vi "p20 codificador imagenes gris.vi"() -> ()   [LabVIEW 2013]
panel:
  in  "path to BMP file 2":path
  in  "path to BMP file":path
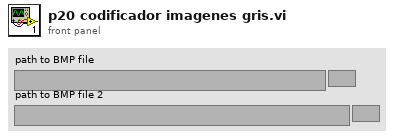
[diagram p1: front panel]
types:
  T1 = typedef "imagedata.ctl" = cluster{"image type":i32, "image depth":i32, "image":u8[], "mask":u8[], "colors":u32[], "Rectangle":cluster{"left":i16, "top":i16, "right":i16, "bottom":i16}}
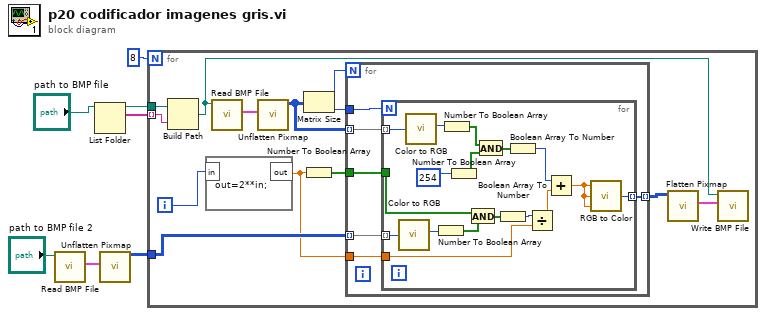
[diagram p0: block diagram]
diagram:
  n1 = call <vilib>:"Read BMP File.vi"("path to BMP file"="path to BMP file 2") -> ("image data"=w2:T1)  [unwired: 8 in, 2 out]
  n2 = List Folder(path="path to BMP file") -> (path out=w5:path, filenames=w4:string[])  [unwired: 3 in, 2 out]
  n3 = call <vilib>:"Unflatten Pixmap.vi"("image data"=w2) -> ("24-bit pixmap"=w1:u32[][])  [unwired: 4 in, 6 out]
  n4 = for {
    N: 8 -> [_]
    tunnel: w5 -> [w19]
    tunnel: w4 -> [w18] mode=indexing
    tunnel: w1 -> [w16]
    i -> [w20]
    n5 = Build Path(base path=w19, name or relative path=w18) -> (appended path=w13:path)
    n6 = formula code="out=2**in;"("in"=w20) -> ("out"=w12:dbl)
    n7 = call <vilib>:"Read BMP File.vi"("path to BMP file"=w13) -> ("image data"=w17:T1)  [unwired: 8 in, 2 out]
    n8 = call <vilib>:"Unflatten Pixmap.vi"("image data"=w17) -> ("24-bit pixmap"=w11:u32[][])  [unwired: 4 in, 6 out]
    n9 = Matrix Size(0:w11) -> (1:w9:i32, 2:w10:i32)
    n10 = Number To Boolean Array(number=w12) -> (Boolean array=w8:bool[])
    n11 = for {
      N: w9 -> [_]
      tunnel: w11 -> [w26] mode=indexing
      tunnel: w16 -> [w25] mode=indexing
      tunnel: [w24] -> w15 mode=indexing
      tunnel: w12 -> [w23]
      tunnel: w10 -> [w22]
      tunnel: w8 -> [w21]
      n12 = for {
        N: w22 -> [_]
        tunnel: w26 -> [w42] mode=indexing
        tunnel: w25 -> [w32] mode=indexing
        tunnel: [w28] -> w24 mode=indexing
        tunnel: w23 -> [w35]
        tunnel: w21 -> [w27]
        n13 = call <vilib>:"Color to RGB.vi"("Color"=w32) -> ("R"=w31:u8)  [unwired: 3 out]
        n14 = call <vilib>:"Color to RGB.vi"("Color"=w42) -> ("R"=w41:u8)  [unwired: 3 out]
        n15 = Number To Boolean Array(number=w31) -> (Boolean array=w30:bool[])
        n16 = Number To Boolean Array(number=w41) -> (Boolean array=w40:bool[])
        n17 = Number To Boolean Array(number=254) -> (Boolean array=w39:bool[])
        n18 = And(x=w27, y=w30) -> (x .and. y?=w37:bool[])
        n19 = And(x=w40, y=w39) -> (x .and. y?=w38:bool[])
        n20 = Boolean Array To Number(Boolean array=w37) -> (number=w34:u32)
        n21 = Boolean Array To Number(Boolean array=w38) -> (number=w36:u32)
        n22 = Divide(x=w34, y=w35) -> (x/y=w29:dbl)
        n23 = Add(x=w36, y=w29) -> (x+y=w33:dbl)
        n24 = call <vilib>:"RGB to Color.vi"("B"=w33, "G"=w33, "R"=w33) -> ("Color"=w28:u32)
      }
    }
    n25 = call <vilib>:"Flatten Pixmap.vi"("24-bit pixmap"=w15) -> ("image data"=w14:T1)  [unwired: 10 in]
    n26 = call <vilib>:"Write BMP File.vi"("image data"=w14, "path to BMP file"=w13) -> ()  [unwired: 8 in, 2 out]
  }
